vi "append_data_h5.vi"(7 "name":string="bg", 8 "error in (no error)":errorcluster, 9 "ref h5_file":T1 format="%.0x", 10 "data":dbl[](array[numeric]), 11 "initialized array":i16[](array[numeric])) -> (0 "error out":errorcluster)   [LabVIEW 2020, in "Detector.lvclass"]
uses:
  Detector.lvclass
  <vilib>/addons/h5labview2/base/hid_t.ctl
  <vilib>/addons/h5labview2/base/lib_path.vi
  <vilib>/addons/h5labview2/base/H5Equery.vi
  <vilib>/addons/h5labview2/dataset/H5Dwrite.llb/H5Dwrite.xnode
  <vilib>/addons/h5labview2/dataset/H5D.lvlib
  <vilib>/addons/h5labview2/space/H5S.lvlib
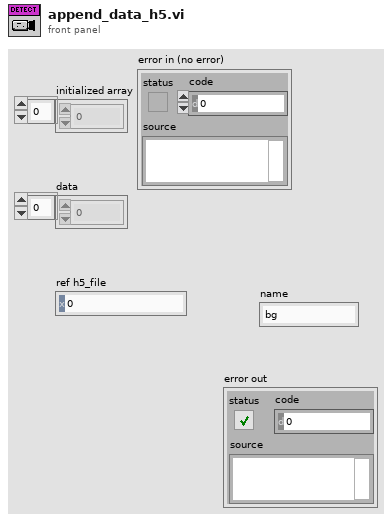
[diagram p1: front panel]
types:
  T1 = typedef "hid_t.ctl" = i64
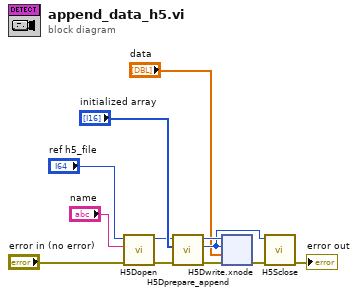
[diagram p0: block diagram]
diagram:
  n1 = call <vilib>:"H5Dopen.vi"("error in (no error)"="error in (no error)", "name"="name", "loc in"="ref h5_file") -> ("error out"=w7:errorcluster, "dset out"=w6:T1)  [unwired: 7 in]
  n2 = call <vilib>:"H5Dprepare_append.vi"("error in (no error)"=w7, "append dims"="initialized array", "dset in"=w6) -> ("error out"=w8:errorcluster, "space out"=w10:T1, "dset out"=w11:T1)  [unwired: 5 in, 1 out]
  n3 = xnode "H5Dwrite.xnode"("error in (no error)"=w8, "data"="data", "file space"=w10, "ref in"=w11) -> ("error out"=w9:errorcluster)  [unwired: 3 in, 2 out]
  n4 = call <vilib>:"H5Sclose.vi"("error in (no error)"=w9, "space in"=w10) -> ("error out"=→"error out":errorcluster)  [unwired: 9 in]
